vi "Write Algo Parameters.vi"(7 "Part Name":string="102", 8 "error in (no error)":errorcluster, 9 "Ticked measurements":i32[](array[numeric])=[0], 10 "Input data cluster":T1={"Tolerance Limits"=[[0.0, 1.0, 0.0, 1.0]], "Measurement Enable"=[TRUE], "Bias Correction"=[0.1], "Linearity Correction"=[0.2]}, 11 "JSON FilePath":path=path "F:/Backup/ZenGage v3.0/20-02-2018/ZenGage v1.1/Configuration file/Algorithm Override JSON.json") -> (0 "error out":errorcluster, 3 "JSON Variant":variant)   [LabVIEW 2015]
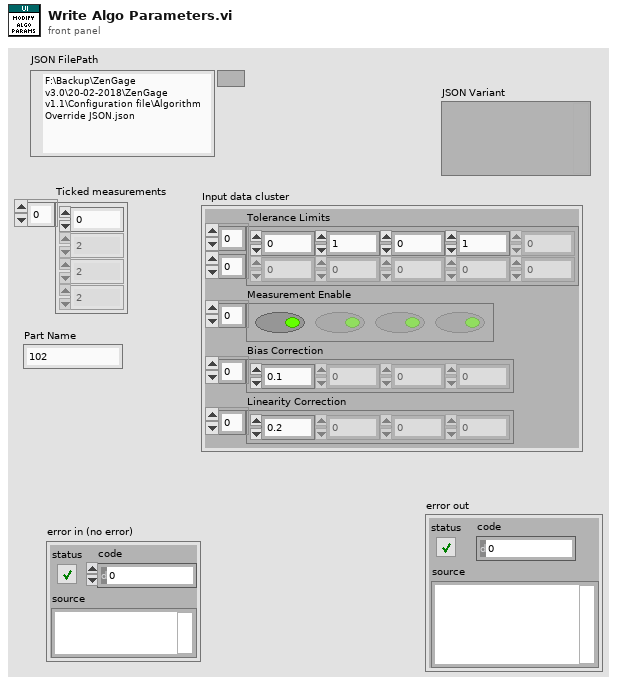
[diagram p1: front panel]
types:
  T1 = cluster{"Tolerance Limits":dbl[][], "Measurement Enable":bool[], "Bias Correction":dbl[], "Linearity Correction":dbl[]}
  T2 = enum16{"Action Failed", "Append", "Insert", "Replace"}
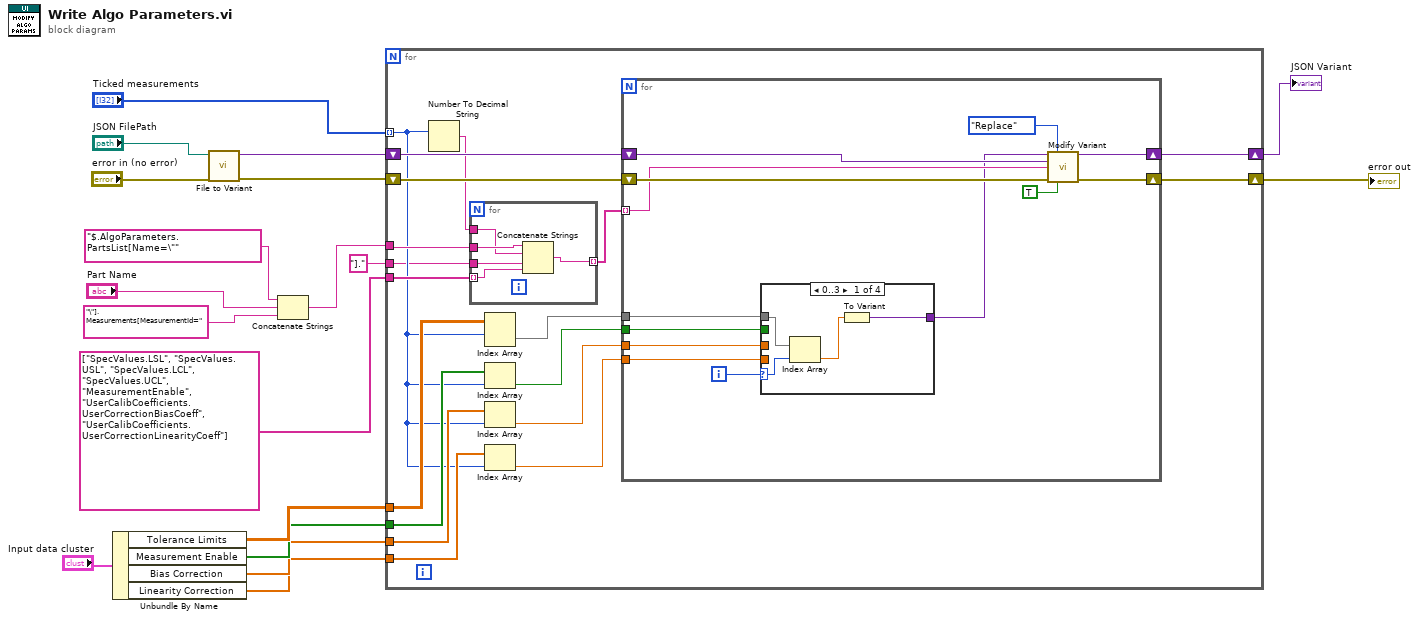
[diagram p0: block diagram]
diagram:
  n1 = Unbundle By Name("Input data cluster") -> ("Tolerance Limits"=w7:dbl[][], "Measurement Enable"=w6:bool[], "Bias Correction"=w5:dbl[], "Linearity Correction"=w4:dbl[])
  n2 = call <vilib>:"File to Variant.vi"("JSON FilePath"="JSON FilePath", "error in (no error)"="error in (no error)") -> ("JSON Variant"=w14:variant, "error out"=w16:errorcluster)  [unwired: 6 in, 1 out]
  n3 = Concatenate Strings("$.AlgoParameters.PartsList[Name=\"", "Part Name", "\"].Measurements[MeasurementId=") -> (w9:string)
  n4 = for {
    tunnel: "Ticked measurements" -> [w22] mode=indexing
    shift-right: [w34] -> w1
    shift-left: w16 -> [w36]
    tunnel: w9 -> [w33]
    tunnel: string[] ["SpecValues.LSL", "SpecValues.USL", "SpecValues.LCL", "SpecValues.UCL", "MeasurementEnable", "UserCalibCoefficients.UserCorrectionBiasCoeff", "UserCalibCoefficients.UserCorrectionLinearityCoeff"] -> [w31]
    shift-right: [w29] -> w3
    shift-left: w14 -> [w35]
    tunnel: w7 -> [w28]
    tunnel: w6 -> [w26]
    tunnel: w5 -> [w24]
    tunnel: w4 -> [w23]
    tunnel: "]." ("string") -> [w19]
    n5 = Number To Decimal String(number=w22) -> (decimal integer string=w32:string)  [unwired: 1 in]
    n6 = for {
      tunnel: w33 -> [w41]
      tunnel: w32 -> [w40]
      tunnel: w31 -> [w38] mode=indexing
      tunnel: [w39] -> w30 mode=indexing
      tunnel: w19 -> [w37]
      n7 = Concatenate Strings(w41, w40, w37, w38) -> (w39:string)
    }
    n8 = Index Array(array=w28, index (row)=w22) -> (element=w27:dbl[])  [unwired: 1 in]
    n9 = Index Array(array=w26, index=w22) -> (element=w25:bool)
    n10 = Index Array(array=w24, index=w22) -> (element=w21:dbl)
    n11 = Index Array(array=w23, index=w22) -> (element=w20:dbl)
    n12 = for {
      shift-right: [w52] -> w34
      shift-left: w36 -> [w54]
      tunnel: w30 -> [w51] mode=indexing
      shift-right: [w48] -> w29
      shift-left: w35 -> [w53]
      tunnel: w27 -> [w42]
      tunnel: w25 -> [w45]
      tunnel: w21 -> [w44]
      tunnel: w20 -> [w43]
      i -> [w47]
      n13 = case shown="0..3" w47 {
        selector: w47 -> [w57 _ _ _]
        tunnel: w42 -> [w56 _ _ _]
        tunnel: [w58 w59 w60 w61] -> w46
        tunnel: w45 -> [_ _ w60 _]
        tunnel: w44 -> [_ _ _ w61]
        tunnel: w43 -> [_ w59 _ _]
        frame 0..3 {
          n14 = Index Array(array=w56, index=w57) -> (element=w55:dbl)
          n15 = To Variant(anything=w55) -> (Variant=w58:variant)
        }
        frame 6 {
        }
        frame 4, Default {
        }
        frame 5 {
        }
      }
      n16 = call <vilib>:"Modify Variant.vi"("New element in"=w46, "Functionality"=T2."Replace", "Parent variant in"=w53, "JSON query path"=w51, "error in (no error)"=w54, "Overwrite\n(Ignore datatype?)"=TRUE ("Overwrite\n(Ignore datatype?)")) -> ("VCluster out"=w48:variant, "error out"=w52:errorcluster)  [unwired: 5 in, 3 out]
    }
  }
  "JSON Variant" <- w3
  "error out" <- w1
